vi "Interp2D.vi"(6 "method":i32(ring)=3 items=["nearest", "bilinear", "bicubic", "bicubic spline"], 7 "Fixed Axis":T1, 9 "Interpolation Points":i32=100, 10 "Meas maxima":dbl[](array[numeric]) format="%.1f", 11 "Measured Points":dbl[][](array[numeric]) format="%.2f") -> (1 "Yi":dbl, 2 "Xi":dbl, 3 "max value":dbl)   [LabVIEW 2022 SP3]
uses:
  <vilib>/Math Plots/3D Math Plots/3D Surface/3D Surface XCtrl/3D Surface.xctl
  Gen Trav/Route mapping/Axis.ctl
  <vilib>/Analysis/1siggen.llb/Ramp Pattern by Samples.vi
  <vilib>/gmath/interp.llb/Create Mesh Grid (2D) (x,y arrays).vi
  <vilib>/gmath/interp.llb/Interpolate 2D (2d X,Y).vi
  <vilib>/Math Plots/3D Math Plots/3D Surface/3D Surface Datatype/Public/Plot Helper (Matrix).vi
  <vilib>/gmath/NI_Gmath.lvlib
  <vilib>/Analysis/NI_AALBase.lvlib
  <vilib>/Math Plots/3D Math Plots/3D Surface/3D Surface Datatype/3D Surface Datatype.lvclass
panel:
  out "Interpolated Surface":refnum<class "3D Plot Datatype.lvclass">[](xcontrol)
  out "Input Surface":refnum<class "3D Plot Datatype.lvclass">[](xcontrol)
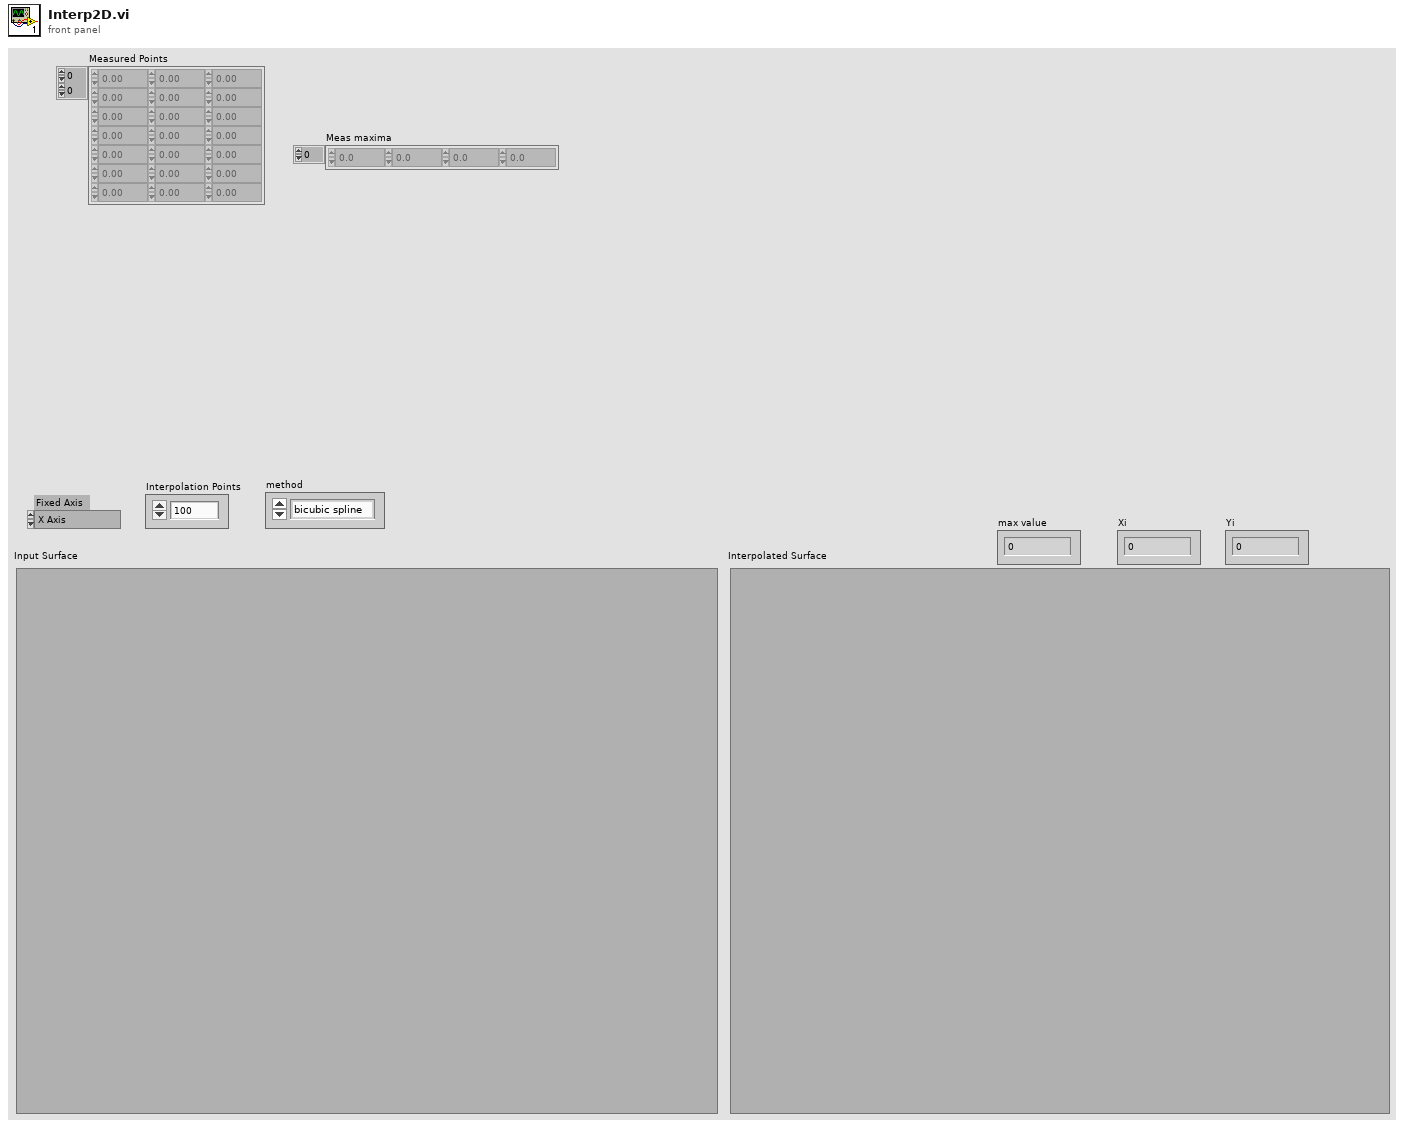
[diagram p1: front panel]
types:
  T1 = typedef "Axis.ctl" = enum16{"X Axis", "X Axis -ve", "Y Axis", "Y Axis -ve", "Z Axis", "Z Axis -ve"}
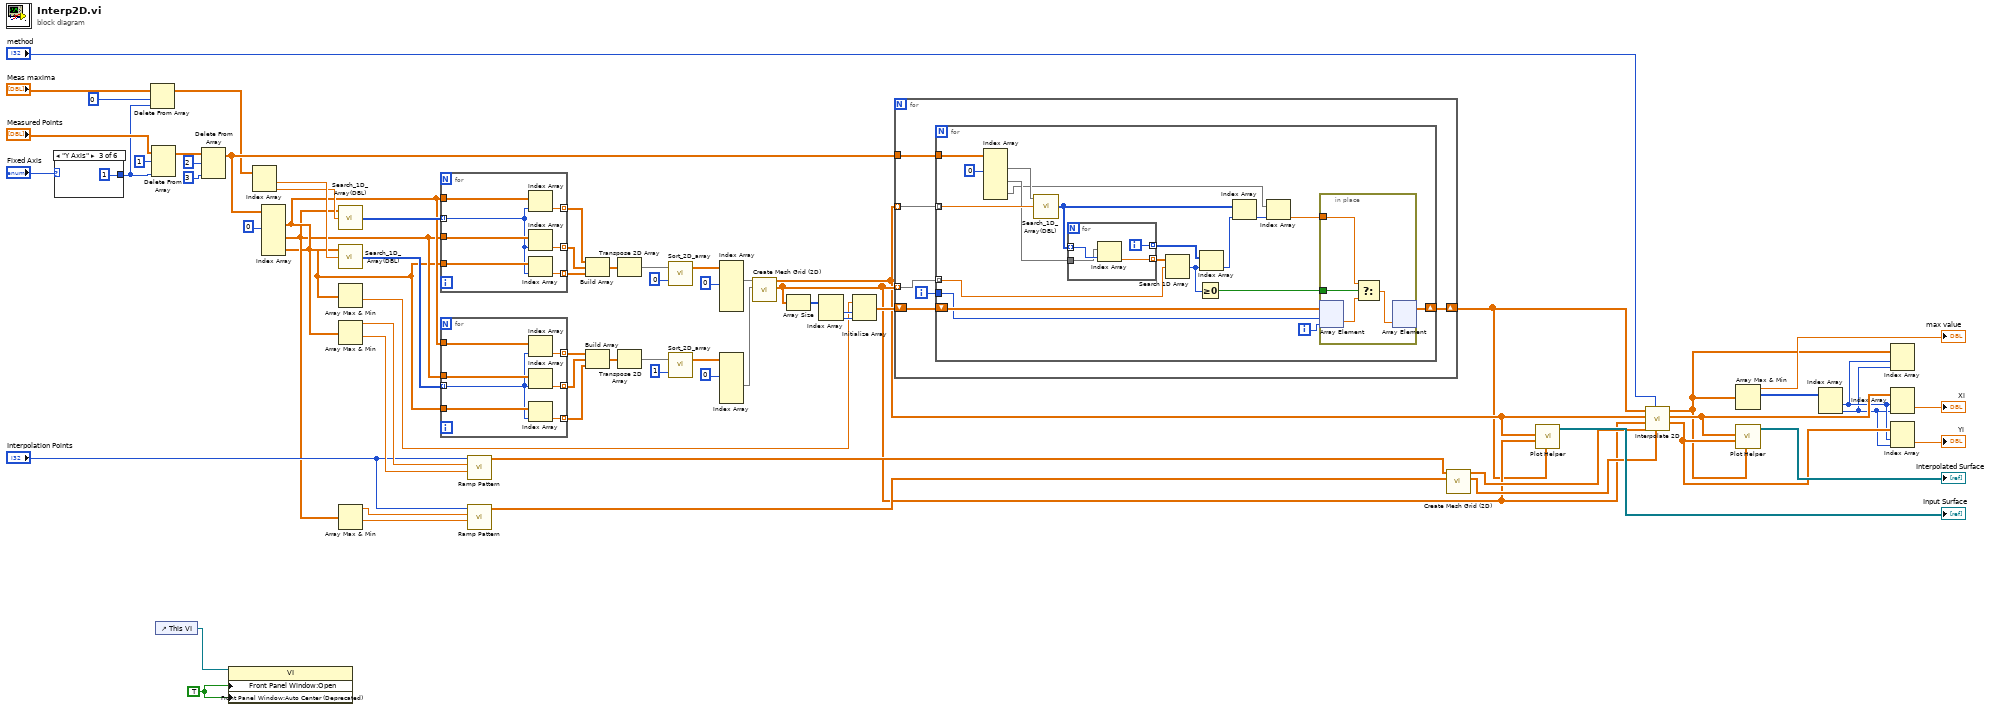
[diagram p0: block diagram]
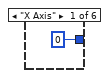
[diagram p2: hidden frame]
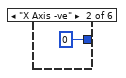
[diagram p3: hidden frame]
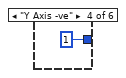
[diagram p4: hidden frame]
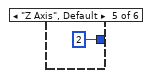
[diagram p5: hidden frame]
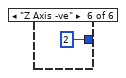
[diagram p6: hidden frame]
diagram:
  w2 = TRUE ("Front Panel Window:Open")
  n1 = case shown="\"Y Axis\"" "Fixed Axis" {
    tunnel: [0 ("index") 0 ("index") 1 ("index") 1 ("index") 2 ("index") 2 ("index")] -> w3
    frame "X Axis" {
    }
    frame "X Axis -ve" {
    }
    frame "Y Axis" {
    }
    frame "Y Axis -ve" {
    }
    frame "Z Axis", Default {
    }
    frame "Z Axis -ve" {
    }
  }
  n2 = Delete From Array(array="Meas maxima", length=0, index=w3) -> (array with subset deleted=w5:dbl[])  [unwired: 1 out]
  n3 = Delete From Array(array="Measured Points", length=1, index (col)=w3) -> (array with subset deleted=w67:dbl[][])  [unwired: 1 in, 1 out]
  n4 = control-ref of="This VI"() -> (w1:refnum<vi>)
  n5 = Delete From Array(array=w67, length=2, index (col)=3 ("disabled index (col)")) -> (array with subset deleted=w18:dbl[][])  [unwired: 1 in, 1 out]
  n6 = property class="VI"(reference=w1, "Front Panel Window:Open"=w2, "Front Panel Window:Auto Center (Deprecated)"=w2) -> ()  [unwired: 1 in, 2 out]
  n7 = Index Array(array=w5) -> (element #1=w57:dbl, element #2=w55:dbl)  [unwired: 2 in]
  n8 = Index Array(array=w18, index (col) #1=0 ("disabled index (col)")) -> (element #1=w43:dbl[], element #2=w42:dbl[], element #3=w17:dbl[])  [unwired: 5 in]
  n9 = call "Search_1D_Array(DBL).vi"("Array"=w42, "Element Data"=w55) -> ("Indicies of Elements"=w54:i32[])  [unwired: 6 in, 1 out]
  n10 = call "Search_1D_Array(DBL).vi"("Array"=w43, "Element Data"=w57) -> ("Indicies of Elements"=w59:i32[])  [unwired: 6 in, 1 out]
  n11 = Array Max & Min(array=w17) -> (min value=w16:dbl)  [unwired: 3 out]
  n12 = Array Max & Min(array=w43) -> (max value=w48:dbl, min value=w47:dbl)  [unwired: 2 out]
  n13 = Array Max & Min(array=w42) -> (max value=w44:dbl, min value=w46:dbl)  [unwired: 2 out]
  n14 = for {
    tunnel: w54 -> [w75] mode=indexing
    tunnel: w43 -> [w81]
    tunnel: w17 -> [w80]
    tunnel: [w79] -> w33 mode=indexing
    tunnel: [w78] -> w52 mode=indexing
    tunnel: [w77] -> w51 mode=indexing
    tunnel: w42 -> [w76]
    n15 = Index Array(array=w81, index=w75) -> (element=w79:dbl)
    n16 = Index Array(array=w76, index=w75) -> (element=w77:dbl)
    n17 = Index Array(array=w80, index=w75) -> (element=w78:dbl)
  }
  n18 = for {
    tunnel: w59 -> [w82] mode=indexing
    tunnel: w43 -> [w88]
    tunnel: w17 -> [w87]
    tunnel: [w86] -> w41 mode=indexing
    tunnel: [w85] -> w56 mode=indexing
    tunnel: [w84] -> w40 mode=indexing
    tunnel: w42 -> [w83]
    n19 = Index Array(array=w88, index=w82) -> (element=w86:dbl)
    n20 = Index Array(array=w83, index=w82) -> (element=w84:dbl)
    n21 = Index Array(array=w87, index=w82) -> (element=w85:dbl)
  }
  n22 = call-poly <vilib>:"Ramp Pattern.vi"("start"=w47, "end"=w48, "samples"="Interpolation Points") -> ("Ramp Pattern"=w27:dbl[])  [unwired: 7 in, 1 out]
  n23 = call-poly <vilib>:"Ramp Pattern.vi"("start"=w46, "end"=w44, "samples"="Interpolation Points") -> ("Ramp Pattern"=w26:dbl[])  [unwired: 7 in, 1 out]
  n24 = Build Array(w33, w51, w52) -> (w53:dbl[][])
  n25 = Build Array(w41, w40, w56) -> (w58:dbl[][])
  n26 = Transpose 2D Array(2D array=w53) -> (transposed array=w49:dbl[][])
  n27 = Transpose 2D Array(2D array=w58) -> (transposed array=w62:dbl[][])
  n28 = call "Sort_2D_array.vi"("Column index to sort on"=0, "unsorted array"=w49) -> ("sorted array"=w34:dbl[][])  [unwired: 1 out]
  n29 = call "Sort_2D_array.vi"("Column index to sort on"=1, "unsorted array"=w62) -> ("sorted array"=w35:dbl[][])  [unwired: 1 out]
  n30 = Index Array(array=w34, index (col) #1=0 ("disabled index (col)")) -> (element #1=w32:dbl[])  [unwired: 5 in, 2 out]
  n31 = Index Array(array=w35, index (col) #1=0 ("disabled index (col)")) -> (element #2=w31:dbl[])  [unwired: 5 in, 2 out]
  n32 = call-poly <vilib>:"Create Mesh Grid (2D).vi"("y domain"=w31, "x domain"=w32) -> ("Y"=w23:dbl[][], "X"=w22:dbl[][])  [unwired: 7 in, 1 out]
  n33 = Array Size(array=w23) -> (size(s)=w39:i32[])
  n34 = Index Array(array=w39) -> (element #1=w38:i32, element #2=w37:i32)  [unwired: 2 in]
  n35 = Initialize Array(w16, w38, w37) -> (w36:dbl[][])
  n36 = for {
    tunnel: w22 -> [w94] mode=indexing
    tunnel: w23 -> [w93] mode=indexing
    tunnel: w18 -> [w92]
    shift-right: [w89] -> w19
    shift-left: w36 -> [w91]
    i -> [w90]
    n37 = for {
      tunnel: w94 -> [w111] mode=indexing
      tunnel: w93 -> [w109] mode=indexing
      tunnel: w92 -> [w113]
      shift-right: [w107] -> w89
      shift-left: w91 -> [w108]
      tunnel: w90 -> [w101]
      i -> [w100]
      n38 = Index Array(array=w113, index (col) #1=0 ("disabled index (col)")) -> (element #1=w110:dbl[], element #2=w106:dbl[], element #3=w104:dbl[])  [unwired: 5 in]
      n39 = call "Search_1D_Array(DBL).vi"("Array"=w110, "Element Data"=w111) -> ("Indicies of Elements"=w96:i32[])  [unwired: 6 in, 1 out]
      n40 = for {
        tunnel: w96 -> [w117] mode=indexing
        tunnel: w106 -> [w116]
        tunnel: [w115] -> w105 mode=indexing
        tunnel: [w114] -> w99 mode=indexing
        i -> [w114]
        n41 = Index Array(array=w116, index=w117) -> (element=w115:dbl)
      }
      n42 = Search 1D Array(1D array=w105, element=w109) -> (index of element=w98:i32)  [unwired: 1 in]
      n43 = Greater Or Equal To 0?(x=w98) -> (x >= 0?=w102:bool)
      n44 = Index Array(array=w99, index=w98) -> (element=w97:i32)
      n45 = Index Array(array=w96, index=w97) -> (element=w95:i32)
      n46 = Index Array(array=w104, index=w95) -> (element=w103:dbl)
      n47 = in-place {
        in-place-border: w103 -> [w120]
        in-place-border: w102 -> [w121]
        n48 = in-place-array #1(w108, w101, w100) -> (w119:dbl)
        n49 = Select(t=w120, s=w121, f=w119) -> (s? t:f=w118:dbl)
        n50 = in-place-array #1(w118) -> (w107:dbl[][])  [unwired: 2 out]
      }
    }
  }
  n51 = call-poly <vilib>:"Create Mesh Grid (2D).vi"("y domain"=w26, "x domain"=w27) -> ("Y"=w24:dbl[][], "X"=w25:dbl[][])  [unwired: 7 in, 1 out]
  n52 = call-poly <vilib>:"Plot Helper.vi"("z matrix"=w19, "y matrix"=w23, "x matrix"=w22) -> ("3D Plot lvclass Array out"=→"Input Surface":refnum<class "3D Plot Datatype.lvclass">[])  [unwired: 3 in, 5 out]
  n53 = call-poly <vilib>:"Interpolate 2D.vi"("yi"=w24, "method"="method", "xi"=w25, "Y"=w23, "X"=w22, "Z"=w19) -> ("yi used"=w13:dbl[][], "xi used"=w14:dbl[][], "zi"=w7:dbl[][])  [unwired: 2 in, 1 out]
  n54 = Array Max & Min(array=w7) -> (max value=→"max value":dbl, max index (indices)=w15:i32[])  [unwired: 2 out]
  n55 = call-poly <vilib>:"Plot Helper.vi"("z matrix"=w7, "y matrix"=w13, "x matrix"=w14) -> ("3D Plot lvclass Array out"=→"Interpolated Surface":refnum<class "3D Plot Datatype.lvclass">[])  [unwired: 3 in, 5 out]
  n56 = Index Array(array=w15) -> (element #1=w9:i32, element #2=w8:i32)  [unwired: 2 in]
  n57 = Index Array(array=w7, index (row)=w9, index (col)=w8) -> ()  [unwired: 1 out]
  n58 = Index Array(array=w14, index (row)=w9, index (col)=w8) -> (element=→"Xi":dbl)
  n59 = Index Array(array=w13, index (row)=w9, index (col)=w8) -> (element=→"Yi":dbl)
